vi "TRDU_TRAMES.vi"(8 "errin":errorcluster, 11 "Go?":bool) -> (0 "errout":errorcluster, 3 "Pass?":bool)   [LabVIEW 2020]
uses:
  <userlib>/PCAN Basic/Controls/BaudrateEenum.ctl
  <userlib>/PCAN Basic/Controls/Channel.ctl
  232ea49e-66b1-4dd1-980e-1338a05048b4.vi
  <userlib>/Alex_Peak_lib/PEAK_lib_ALEX.lvlib
  <userlib>/PCAN Basic/PCANBasic.lvlib
panel:
  out "Roll_Counter_u8":bool
  out "Array 2":dbl[](array[numeric])
  out "Waveform Chart":dbl(graph)
  out "Array":T1(array[cluster]) {"ID" format="%.0x"}
  out "Numeric":i32
  out "Température (°C) 2":dbl
  out "Min":dbl=100.0
  out "Max":dbl=-100.0
  in  "TRDU CLUSTER IN":T2
  in  "Stop":bool
  # "Voir conversion"
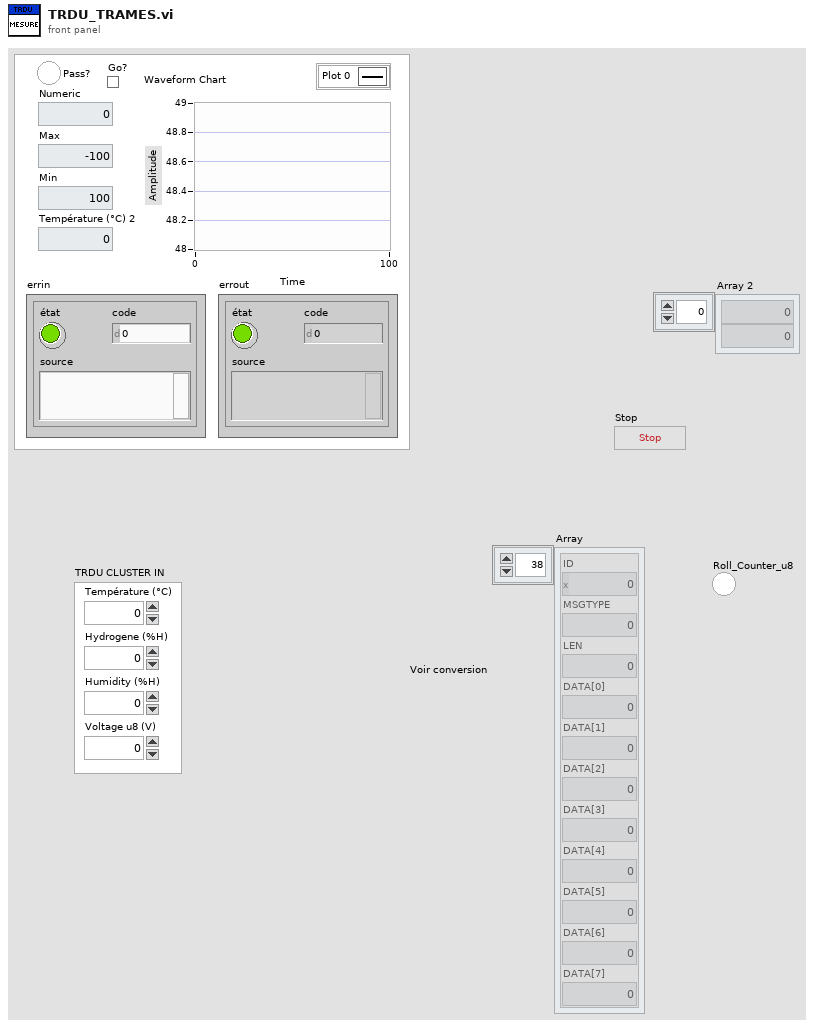
[diagram p1: front panel]
types:
  T1 = cluster{"ID":u32, "MSGTYPE":u8, "LEN":u8, "DATA[0]":u8, "DATA[1]":u8, "DATA[2]":u8, "DATA[3]":u8, "DATA[4]":u8, "DATA[5]":u8, "DATA[6]":u8, "DATA[7]":u8}[]
  T2 = cluster{"Température (°C)":dbl, "Hydrogene (%H)":dbl, "Humidity (%H)":dbl, "Voltage u8 (V)":dbl}
  T3 = typedef "PCANBasic.lvlib/Channel.ctl" = enum16{"PCAN_NONEBUS", "not used1", "not used2", "not used3", "not used4", "not used5", "not used6", "not used7", "not used8", "not used9", "not used10", "not used11", "not used12", "not used13", "not used14", "not used15", "not used16", "not used17", "not used18", "not used19", "not used20", "not used21", "not used22", "not used23", "not used24", "not used25", "not used26", "not used27", "not used28", "not used29", "not used30", "not used31", "not used32", "PCAN_ISABUS1", "PCAN_ISABUS2", "PCAN_ISABUS3", "PCAN_ISABUS4", "PCAN_ISABUS5", "PCAN_ISABUS6", "PCAN_ISABUS7", "PCAN_ISABUS8", "not used41", "not used42", "not used43", "not used44", "not used45", "not used46", "not used47", "not used48", "PCAN_DNGBUS1", "not used50", "not used51", "not used52", "not used53", "not used54", "not used55", "not used56", "not used57", "not used58", "not used59", "not used60", "not used61", "not used62", "not used63", "not used64", "PCAN_PCIBUS1", "PCAN_PCIBUS2", "PCAN_PCIBUS3", "PCAN_PCIBUS4", "PCAN_PCIBUS5", "PCAN_PCIBUS6", "PCAN_PCIBUS7", "PCAN_PCIBUS8", "not used73", "not used74", "not used75", "not used76", "not used77", "not used78", "not used79", "not used80", "PCAN_USBBUS1", "PCAN_USBBUS2", "PCAN_USBBUS3", "PCAN_USBBUS4", "PCAN_USBBUS5", "PCAN_USBBUS6", "PCAN_USBBUS7", "PCAN_USBBUS8", "Not used89", "Not used90", "Not used91", "Not used92", "Not used93", "Not used94", "Not used95", "Not used96", "PCAN_PCCBUS1", "PCAN_PCCBUS2"}
  T4 = typedef "PCANBasic.lvlib/BaudrateEenum.ctl" = enum16{"CAN_Baud_1M", "CAN_Baud_800K", "CAN_BAUD_500K", "CAN_BAUD_250K", "CAN_BAUD_125K", "CAN_BAUD_100K", "CAN_BAUD_95K", "CAN_BAUD_83K", "CAN_BAUD_50K", "CAN_BAUD_47K", "CAN_BAUD_33K", "CAN_BAUD_20K", "CAN_BAUD_10K", "CAN_BAUD_5K", "User Baudrate"}
  T5 = cluster{"ID":u32, "MSGTYPE":u8, "LEN":u8, "DATA[0]":u8, "DATA[1]":u8, "DATA[2]":u8, "DATA[3]":u8, "DATA[4]":u8, "DATA[5]":u8, "DATA[6]":u8, "DATA[7]":u8}
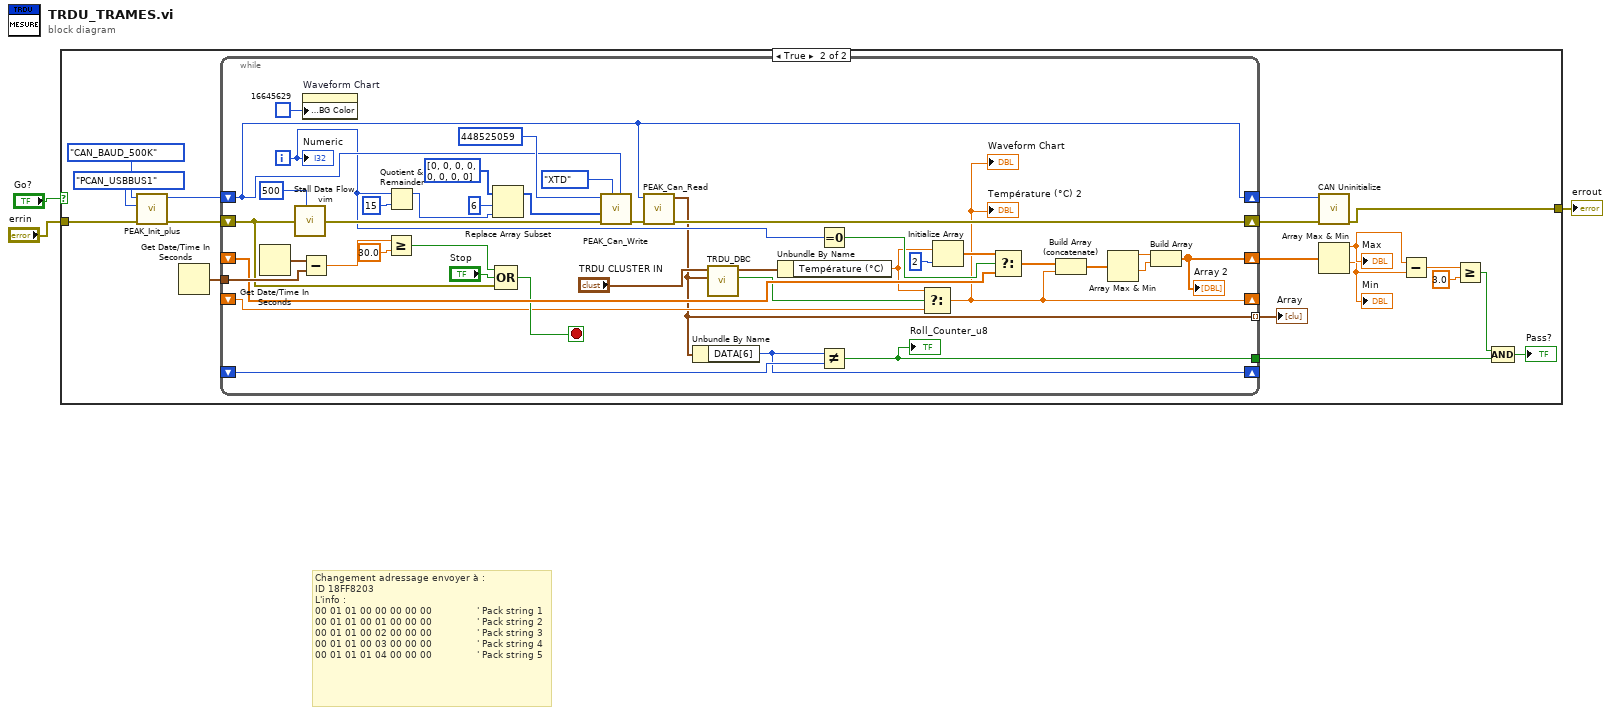
[diagram p0: block diagram]
diagram:
  # "Changement adressage envoyer à :\nID 18FF8203 \nL'info :\n00 01 01 00 00 00 00 00               ' Pack string 1\n00 01 01 00 01 00 00 00               ' Pack string 2\n00 01 01 00 02 00 00 00               ' Pack string 3\n00 01 01 00 03 00 00 00               ' Pack string 4\n00 01 01 01 04 00 00 00               ' Pack string 5"
  n1 = case shown="True" "Go?" {
    tunnel: "errin" -> [w4 w6]
    tunnel: [w4 w5] -> w1
    frame False {
    }
    frame True {
      n2 = call <userlib>:"PEAK_Init_plus.vi"("errin"=w6, "Channel"=Channel."PCAN_USBBUS1", "BTR0BTR1"=BaudrateEenum."CAN_BAUD_500K") -> ("errout"=w22:errorcluster, "Channel out"=w19:T3)  [unwired: 7 in]
      n3 = Get Date/Time In Seconds() -> (seconds since 1Jan1904=w18:timestamp)
      n4 = while {
        shift-right: [w61] -> w20
        shift-left: w22 -> [w34]
        tunnel: w18 -> [w48]
        shift-right: [w47] -> w17
        shift-left: w19 -> [w47]
        shift-right: [w43] -> w16
        shift-left: _ -> [w37]
        tunnel: [w25] -> w15 mode=indexing
        shift-right: [w28] -> _
        shift-left: _ -> [w29]
        shift-right: [w24] -> _
        shift-left: _ -> [w27]
        tunnel: [w26] -> w13
        i -> [w41]
        stop <- w33 stop-if-true
        n5 = Get Date/Time In Seconds() -> (seconds since 1Jan1904=w49:timestamp)
        n6 = call "Stall Data Flow.vim"("value in"=w34, "milliseconds to wait"=u32 500) -> ("value out"=w56:errorcluster)  [unwired: 1 out]
        n7 = Subtract(x=w49, y=w48) -> (x-y=w51:dbl)
        n8 = property on="Waveform Chart" class="WFChart (strict)"("Plot Area:Colors:BG Color"=u32 16645629) -> ()  [unwired: 2 in, 2 out]
        n9 = Greater Or Equal?(x=w51, y=30.0) -> (x >= y?=w36:bool)
        n10 = Quotient & Remainder(x=w41, y=15) -> (x-y*floor(x/y)=w60:i32)  [unwired: 1 out]
        n11 = Replace Array Subset(array=u8[] [0, 0, 0, 0, 0, 0, 0, 0] ("CAN Data"), new element=w60, index=6 ("indice")) -> (w54:u8[])
        n12 = Compound Arithmetic op=OR(w36, "Stop", w34) -> (w33:bool)
        n13 = call <userlib>:"PEAK_Can_Write.vi"("CAN handle"=w47, "MSG type"=enum8{"STD", "RTR", "XTD", "XTD RTR", "STATUS"}."XTD", "errin"=w56, "CAN Data"=w54, "Identifier"=u32 448525059) -> ("errout"=w63:errorcluster)  [unwired: 6 in]
        n14 = call <userlib>:"PEAK_Can_Read.vi"("errin"=w63, "Channel out"=w47) -> ("errout"=w61:errorcluster, "MessageBuffer out"=w25:T5)  [unwired: 7 in, 1 out]
        n15 = Unbundle By Name(w25) -> ("DATA[6]"=w24:u8)
        n16 = call "TRDU_DBC.vi"("Datain"=w25, "TRDU CLUSTER IN in"="TRDU CLUSTER IN") -> ("x = y?"=w31:bool, "TRDU CLUSTER IN out"=w52:T2)  [unwired: 8 in]
        n17 = Unbundle By Name(w52) -> ("Température (°C)"=w30:dbl)
        n18 = Equal To 0?(x=w41) -> (x = 0?=w42:bool)
        n19 = Not Equal?(x=w24, y=w27) -> (x != y?=w26:bool)
        "Roll_Counter_u8" <- w26
        n20 = Select(t=w30, s=w31, f=w29) -> (s? t:f=w28:dbl)
        "Température (°C) 2" <- w28
        "Waveform Chart" <- w28
        n21 = Initialize Array(w30, 2 ("dimension size")) -> (w39:dbl[])
        n22 = Select(t=w39, s=w42, f=w37) -> (s? t:f=w38:dbl[])
        n23 = Build Array (concatenate)(w38, w28) -> (w44:dbl[])
        n24 = Array Max & Min(array=w44) -> (max value=w46:dbl, min value=w45:dbl)  [unwired: 2 out]
        n25 = Build Array(w46, w45) -> (w43:dbl[])
        "Array 2" <- w43
        "Numeric" <- w41
      }
      "Array" <- w15
      n26 = call <userlib>:"CAN Uninitialize.vi"("error in (no error)"=w20, "Channel"=w17) -> ("error out"=w5:errorcluster)  [unwired: 7 in, 2 out]
      n27 = Array Max & Min(array=w16) -> (max value=w12:dbl, min value=w11:dbl)  [unwired: 2 out]
      "Max" <- w12
      "Min" <- w11
      n28 = Subtract(x=w12, y=w11) -> (x-y=w10:dbl)
      n29 = Greater Or Equal?(x=w10, y=3.0) -> (x >= y?=w8:bool)
      n30 = Compound Arithmetic op=AND(w8, w13) -> (→"Pass?":bool)
    }
  }
  "errout" <- w1
